vi "Send_Multiple_Event.vi"(7 "cmd":string[](array[string]), 8 "Error in":errorcluster, 9 "Data":variant[](array[variant]), 11 "User Event in":refnum<user-event>) -> (0 "Error out":errorcluster, 3 "User Event":refnum<user-event>)   [LabVIEW 2021]
uses:
  typedef/Queue_Cluster.ctl
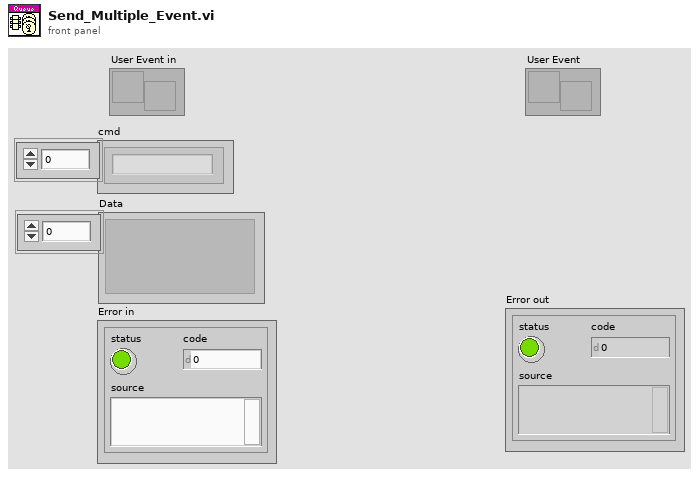
[diagram p1: front panel]
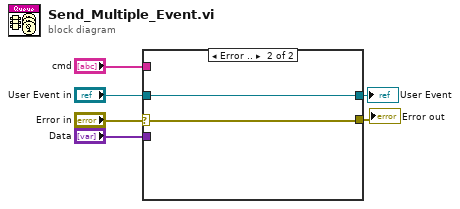
[diagram p0: block diagram]
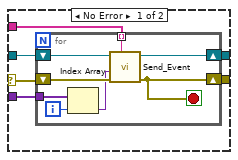
[diagram p2: hidden frame]
diagram:
  n1 = case shown="Error .." "Error in" {
    selector: "Error in" -> [w7 w22]
    tunnel: "User Event in" -> [w12 w21]
    tunnel: "cmd" -> [w11 _]
    tunnel: "Data" -> [w10 _]
    tunnel: [w9 w21] -> w3
    tunnel: [w8 w22] -> w2
    frame No Error {
      n2 = for {
        shift-right: [w19] -> w9
        shift-left: w12 -> [w20]
        shift-right: [w13] -> w8
        shift-left: w7 -> [w18]
        tunnel: w11 -> [w17] mode=indexing
        tunnel: w10 -> [w16]
        i -> [w15]
        stop <- w13 stop-if-true
        n3 = Index Array(array=w16, index=w15) -> (element=w14:variant)
        n4 = call "Send_Event.vi"("cmd"=w17, "Error in"=w18, "Data"=w14, "User Event in"=w20) -> ("error out"=w13:errorcluster, "User Event out"=w19:refnum<user-event>)  [unwired: 6 in]
      }
    }
    frame Error {
    }
  }
  "User Event" <- w3
  "Error out" <- w2
